vi "StockFPGA_InlinedWaitFor1OrMoreIRQs.vi"(0 "session in":T1, 5 "interrupt base address":u32 format="%.0x", 7 "interrupt number(s) mask":u32 format="%.0x", 9 "timeout in ms (-1 for no timeout)":i32, 11 "error in (no error)":errorcluster) -> (4 "session out":T1, 6 "status register if irq received":u32, 8 "timed out?":bool, 10 "interrupt received?":bool, 15 "error out":errorcluster)   [LabVIEW 2022 SP3]
uses:
  niFpgaHostInterfaceSession.ctl
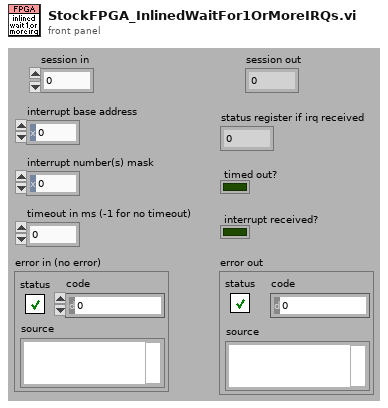
[diagram p1: front panel]
types:
  T1 = typedef "niFpgaHostInterfaceSession.ctl" = u32
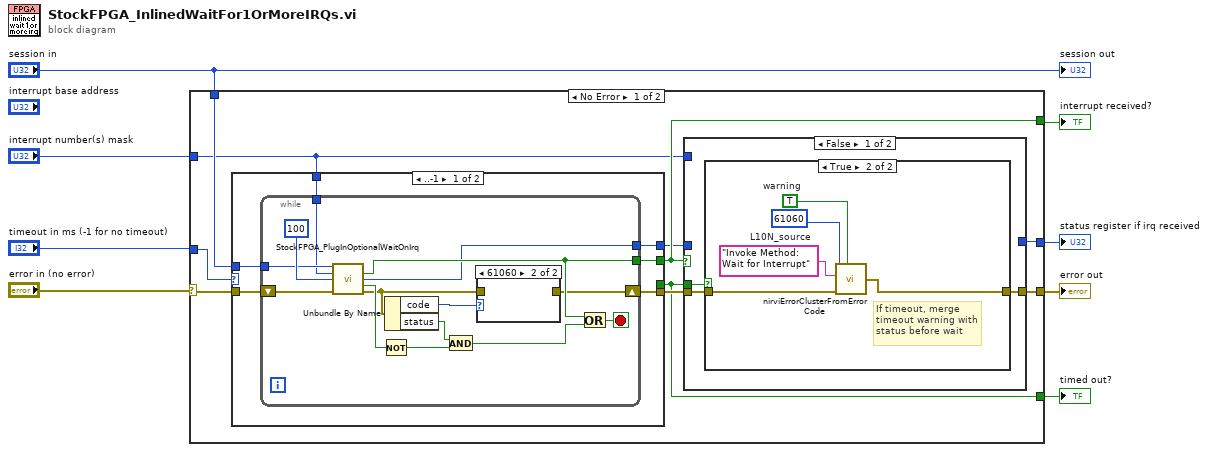
[diagram p0: block diagram]
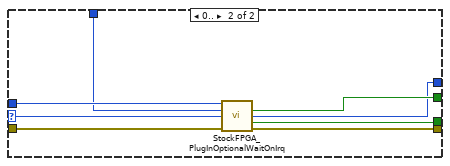
[diagram p3: hidden frame]
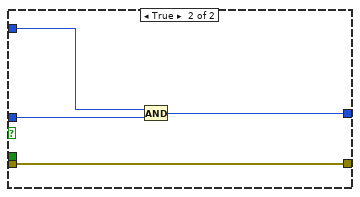
[diagram p5: hidden frame]
diagram:
  n1 = case shown="No Error" "error in (no error)" {
    selector: "error in (no error)" -> [w12 w61]
    tunnel: "session in" -> [w11 _]
    tunnel: "interrupt number(s) mask" -> [w9 _]
    tunnel: [w18 w61] -> w7
    tunnel: [w16 _] -> w6
    tunnel: "timeout in ms (-1 for no timeout)" -> [w15 _]
    tunnel: [w14 _] -> w8
    tunnel: [w13 _] -> w5
    frame No Error {
      n2 = case shown="..-1" w15 {
        selector: w15 -> [_ w44]
        tunnel: [w21 w46] -> w13
        tunnel: w11 -> [w24 w42]
        tunnel: w12 -> [w23 w43]
        tunnel: [w22 w47] -> w17
        tunnel: [_ w45] -> w16
        tunnel: w9 -> [w19 w41]
        tunnel: [w20 w40] -> w10
        frame ..-1 {
          n3 = while {
            tunnel: w24 -> [w33]
            tunnel: [w36] -> w21
            shift-right: [w25] -> w22
            shift-left: w23 -> [w34]
            tunnel: [w30] -> w20
            tunnel: w19 -> [w29]
            stop <- w38 stop-if-true
            n4 = call "StockFPGA_PlugInOptionalWaitOnIrq.vi"("session in"=w33, "interrupt number(s) mask"=w29, "timeout in ms"=100 ("timeout (0)"), "error in (no error)"=w34) -> ("interrupt received?"=w36:bool, "status register if irq received"=w30:u32, "timed out?"=w32:bool, "error out"=w26:errorcluster)  [unwired: 7 in, 1 out]
            n5 = Not(x=w32) -> (.not. x?=w31:bool)
            n6 = Unbundle By Name(w26) -> ("code"=w27:i32, "status"=w28:bool)
            n7 = And(x=w28, y=w31) -> (x .and. y?=w37:bool)
            n8 = case shown="61060" w27 {
              tunnel: w26 -> [w39 _]
              tunnel: [w39 _] -> w25
              frame Default {
              }
              frame 61060 {
              }
            }
            n9 = Or(x=w36, y=w37) -> (x .or. y?=w38:bool)
          }
        }
        frame 0.. {
          n10 = call "StockFPGA_PlugInOptionalWaitOnIrq.vi"("session in"=w42, "interrupt number(s) mask"=w41, "timeout in ms"=w44, "error in (no error)"=w43) -> ("interrupt received?"=w46:bool, "status register if irq received"=w40:u32, "timed out?"=w45:bool, "error out"=w47:errorcluster)  [unwired: 7 in, 1 out]
        }
      }
      n11 = case shown="False" w13 {
        tunnel: [w49 w60] -> w18
        tunnel: w17 -> [w50 w60]
        tunnel: w9 -> [_ w59]
        tunnel: w16 -> [w48 _]
        tunnel: [_ w57] -> w14
        tunnel: w10 -> [_ w58]
        frame False {
          n12 = case shown="True" w48 {
            tunnel: w50 -> [w51 w53]
            tunnel: [w51 w52] -> w49
            frame False {
            }
            frame True {
              w55 = TRUE  # warning
              w54 = "Invoke Method: Wait for Interrupt"  # L10N_source
              # "If timeout, merge timeout warning with status before wait"
              n13 = call <vilib>:"nirviErrorClusterFromErrorCode.vi"("error code"=61060 ("code"), "Function Name"=w54, "error in"=w53, "warning"=w55) -> ("error out"=w52:errorcluster)  [unwired: 1 in]
            }
          }
        }
        frame True {
          n14 = And(x=w59, y=w58) -> (x .and. y?=w57:u32)
        }
      }
    }
    frame Error {
    }
  }
  "timed out?" <- w6
  "error out" <- w7
  "interrupt received?" <- w5
  "status register if irq received" <- w8
  "session out" <- "session in"
